vi "_AMI.vi"(1 "输入":i8[](array[numeric])) -> (0 "输出":i8[](array[numeric]))   [LabVIEW 2018]
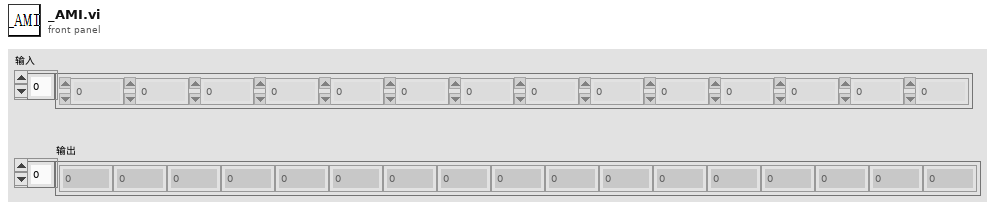
[diagram p1: front panel]
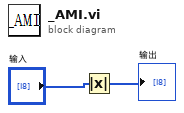
[diagram p0: block diagram]
diagram:
  n1 = Absolute Value(x="输入") -> (abs(x)=→"输出":i8[])
